vi "Coord window-Save as.vi"(11 "file path":path) -> (0 "error out":errorcluster)   [LabVIEW 2020]
uses:
  Globals/Coord window-Globals.vi
  <userlib>/My Palettes.lib/Files & paths/Spreadsheet/Write To Spreadsheet File (string)-Mod.vi
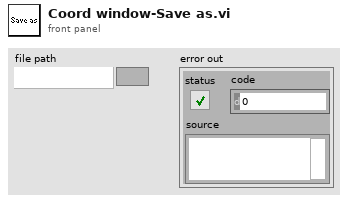
[diagram p1: front panel]
types:
  T1 = typedef "Coordinate list window refs.ctl" = cluster{"Window Name (i.e. Key)":string, "menu reference":refnum<k9>, "VI's reference":refnum<vi>, "Pane 1":refnum<vi>, "Pane 2":refnum<vi>, "Coord Listbox":refnum<vi>, "File name":refnum<vi>, "Picture Map":refnum<vi>, "Stage XYZ Position ind.":refnum<vi>}
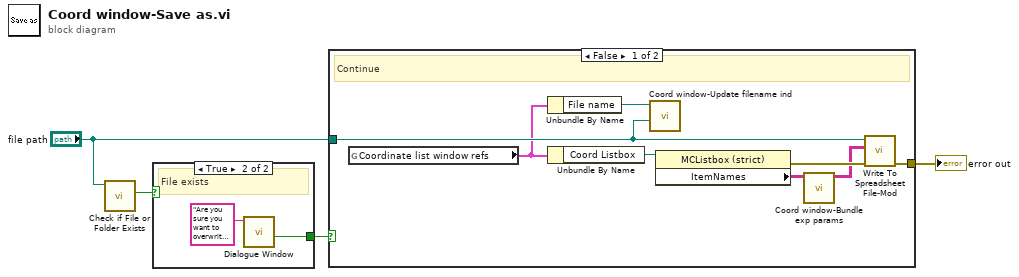
[diagram p0: block diagram]
diagram:
  n1 = call <vilib>:"Check if File or Folder Exists.vi"("path"="file path") -> ("file or folder exists?"=w4:bool)  [unwired: 8 in, 2 out]
  n2 = case shown="True" w4 {
    tunnel: [_ w5] -> w2
    frame False {
      # "File doens't already exist"
    }
    frame True {
      # "File exists"
      n3 = call "Dialogue Window.vi"("Message string"="Are you sure you want to overwrite the existing file?") -> ("Cancelled (Left button pressed)"=w5:bool)  [unwired: 8 in, 2 out]
    }
  }
  n4 = case shown="False" w2 {
    tunnel: [w11 _] -> w3
    tunnel: "file path" -> [w10 _]
    frame False {
      # "Continue"
      n5 = global read "Coord window-Globals.vi" "Coordinate list window refs"() -> (w9:T1)
      n6 = Unbundle By Name(w9) -> ("File name"=w14:refnum<vi>)
      n7 = Unbundle By Name(w9) -> ("Coord Listbox"=w13:refnum<vi>)
      n8 = call "Coord window-Update filename ind.vi"("File path"=w10, "File name indicator ref"=w14) -> ()  [unwired: 9 in, 1 out]
      n9 = property on="Property Node" class="MCListbox (strict)"(reference=w13) -> (error out=w12:errorcluster, "ItemNames"=w8:string[][])  [unwired: 1 in, 1 out]
      n10 = call "Coord window-Bundle exp params.vi"("Item Names"=w8) -> ("Item Names + exp params"=w7:string[][])  [unwired: 10 in]
      n11 = call-poly <userlib>:"Write To Spreadsheet File-Mod.vi"("error in"=w12, "2D data"=w7, "file path (dialog if empty)"=w10) -> ("error out"=w11:errorcluster)  [unwired: 7 in, 1 out]
    }
    frame True {
      # "Cancelled"
    }
  }
  "error out" <- w3
